vi "Get All Children of a Parent.vi"(8 "Error In":errorcluster, 10 "Parent tag":string, 11 "Tree ref":refnum<vi>) -> (0 "Error out":errorcluster, 1 "All Children":string[](array[string]), 2 "Parent tag out":string, 3 "Tree ref out":refnum<vi>)   [LabVIEW 2018]
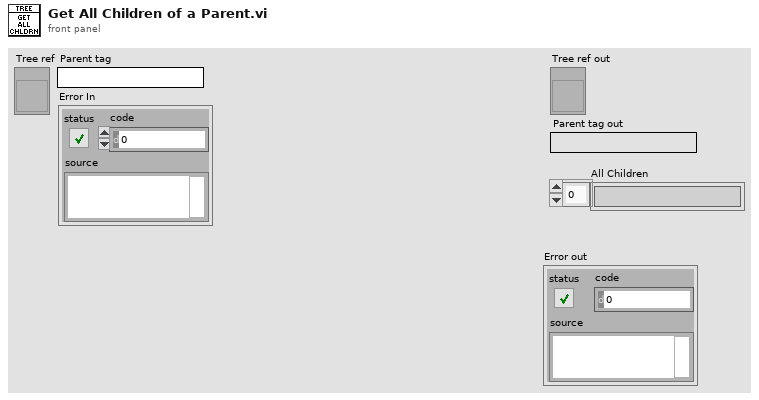
[diagram p1: front panel]
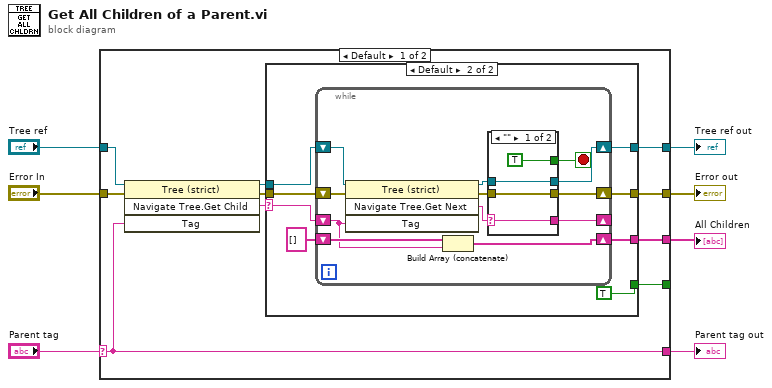
[diagram p0: block diagram]
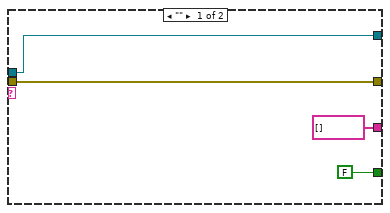
[diagram p2: hidden frame]
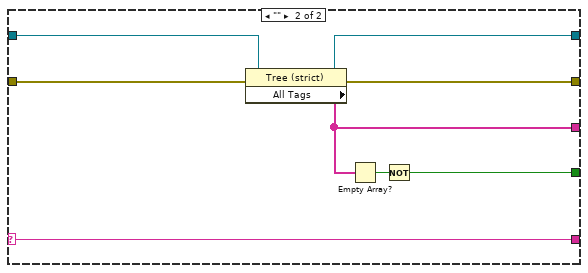
[diagram p4: hidden frame]
diagram:
  n1 = case shown="Default" "Parent tag" {
    selector: "Parent tag" -> [w8 w52]
    tunnel: [w17 w51] -> w4
    tunnel: [w16 w54] -> w2
    tunnel: "Error In" -> [w15 w56]
    tunnel: "Tree ref" -> [w14 w55]
    tunnel: [w11 w53] -> w3
    tunnel: [w9 w49] -> _
    tunnel: [w8 w52] -> w1
    frame Default {
      n2 = invoke class="Tree (strict)" method="Navigate Tree.Get Child"(reference=w14, error in=w15, "Tag"=w8) -> (reference out=w13:refnum<vi>, error out=w12:errorcluster, "Navigate Tree:Get Child"=w10:string)  [unwired: 1 in, 1 out]
      n3 = case shown="Default" w10 {
        selector: w10 -> [_ w23]
        tunnel: [string[] [] w29] -> w17
        tunnel: [w20 w28] -> w16
        tunnel: w13 -> [w21 w27]
        tunnel: w12 -> [w20 w26]
        tunnel: [w21 w25] -> w11
        tunnel: [FALSE ("Children Found?") TRUE ("Children Found?")] -> w9
        frame "" {
        }
        frame Default {
          n4 = while {
            shift-right: [w36] -> w28
            shift-left: w26 -> [w41]
            shift-right: [w37] -> w25
            shift-left: w27 -> [w40]
            shift-right: [w35] -> _
            shift-left: w23 -> [w30]
            shift-right: [w31] -> w29
            shift-left: string[] [] -> [w32]
            stop <- w33 stop-if-true
            n5 = invoke class="Tree (strict)" method="Navigate Tree.Get Next"(reference=w40, error in=w41, "Tag"=w30) -> (reference out=w38:refnum<vi>, error out=w39:errorcluster, "Navigate Tree:Get Next Item"=w34:string)  [unwired: 1 in, 1 out]
            n6 = Build Array (concatenate)(w32, w30) -> (w31:string[])
            n7 = case shown="\"\"" w34 {
              selector: w34 -> [w42 w46]
              tunnel: w39 -> [w45 w47]
              tunnel: w38 -> [w44 w48]
              tunnel: [w44 w48] -> w37
              tunnel: [w45 w47] -> w36
              tunnel: [w42 w46] -> w35
              tunnel: [TRUE _] -> w33
              frame "" {
              }
              frame Default {
              }
            }
          }
        }
      }
    }
    frame "" {
      n8 = property class="Tree (strict)"(reference=w55, error in=w56) -> (reference out=w53:refnum<vi>, error out=w54:errorcluster, "All Tags"=w51:string[])
      n9 = Empty Array?(array=w51) -> (empty?=w50:bool)
      n10 = Not(x=w50) -> (.not. x?=w49:bool)
    }
  }
  "Tree ref out" <- w3
  "Parent tag out" <- w1
  "All Children" <- w4
  "Error out" <- w2
